vi "PC_SetSelectResistorTo_PLC.vi"(0 "VISA resource name":refnum<visa-resource-name>, 1 "Mode":enum16{"RTU", "ASCII"}(ring), 2 "PLC Address":u8, 3 "Resistor":i32, 5 "error in (no error)":errorcluster) -> (6 "VISA resource name out":refnum<visa-resource-name>, 8 "error out":errorcluster)   [LabVIEW 2015]
panel:
  out "Array":i32[](array[numeric])
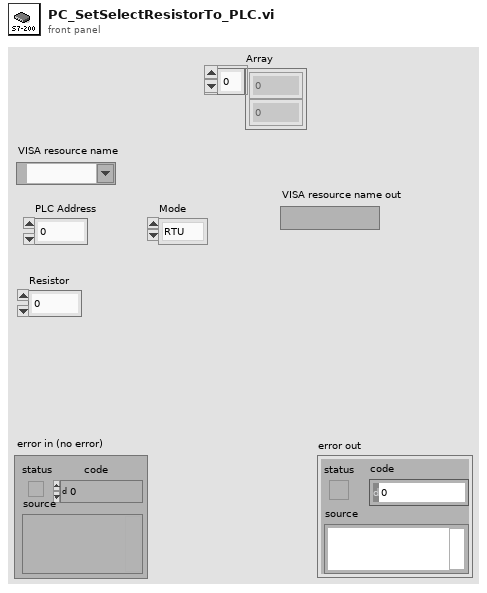
[diagram p1: front panel]
types:
  T1 = cluster{"Mode":enum16{"RTU", "ASCII"}, "Slave Address":u8}
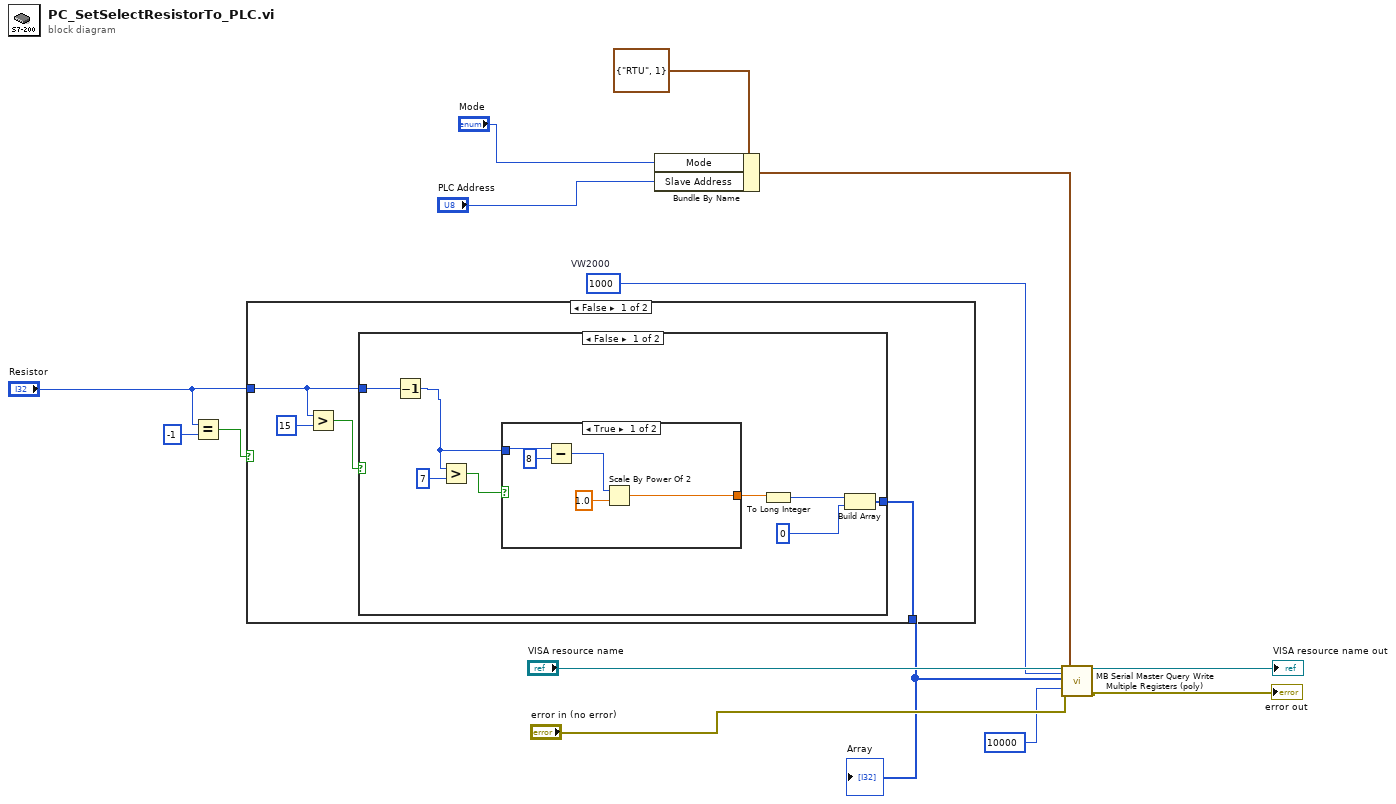
[diagram p0: block diagram]
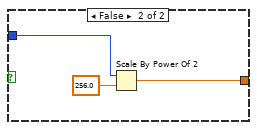
[diagram p2: hidden frame]
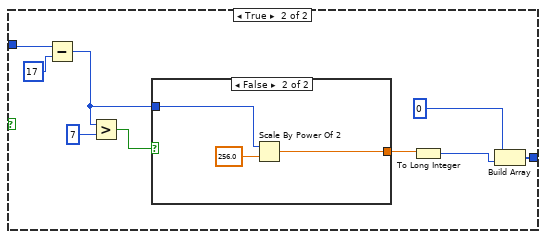
[diagram p3: hidden frame]
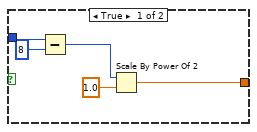
[diagram p4: hidden frame]
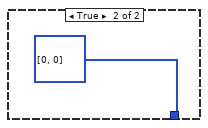
[diagram p5: hidden frame]
diagram:
  w5 = u16 1000  # VW2000
  n1 = Equal?(x="Resistor", y=-1) -> (x = y?=w2:bool)
  n2 = case shown="False" w2 {
    tunnel: "Resistor" -> [w16 _]
    tunnel: [w15 i32[] [0, 0]] -> w4
    frame False {
      n3 = Greater?(x=w16, y=15) -> (0:w17:bool)
      n4 = case shown="False" w17 {
        tunnel: w16 -> [w20 w37]
        tunnel: [w21 w40] -> w15
        frame False {
          n5 = Decrement(x=w20) -> (x-1=w19:i32)
          n6 = Greater?(x=w19, y=7) -> (0:w25:bool)
          n7 = case shown="True" w25 {
            tunnel: w19 -> [w29 w33]
            tunnel: [w30 w32] -> w24
            frame True {
              n8 = Subtract(x=w29, y=8) -> (x-y=w27:i32)
              n9 = Scale By Power Of 2(n=w27, x=1.0) -> (x*2^n=w30:dbl)
            }
            frame False {
              n10 = Scale By Power Of 2(n=w33, x=256.0) -> (x*2^n=w32:dbl)
            }
          }
          n11 = To Long Integer(number=w24) -> (32bit integer=w23:i32)
          n12 = Build Array(w23, 0) -> (w21:i32[])
        }
        frame True {
          n13 = Subtract(x=w37, y=17) -> (x-y=w35:i32)
          n14 = Greater?(x=w35, y=7) -> (0:w42:bool)
          n15 = case shown="False" w42 {
            tunnel: w35 -> [w46 w50]
            tunnel: [w47 w49] -> w41
            frame True {
              n16 = Subtract(x=w46, y=8) -> (x-y=w44:i32)
              n17 = Scale By Power Of 2(n=w44, x=1.0) -> (x*2^n=w47:dbl)
            }
            frame False {
              n18 = Scale By Power Of 2(n=w50, x=256.0) -> (x*2^n=w49:dbl)
            }
          }
          n19 = To Long Integer(number=w41) -> (32bit integer=w39:i32)
          n20 = Build Array(0, w39) -> (w40:i32[])
        }
      }
    }
    frame True {
    }
  }
  "Array" <- w4
  n21 = Bundle By Name(cluster=T1 {"Mode"=enum."RTU", "Slave Address"=1} ("Serial Parameters"), "Mode"="Mode", "Slave Address"="PLC Address") -> (w8:T1)
  n22 = call "MB Serial Master Query Write Multiple Registers (poly).vi"("VISA resource name"="VISA resource name", "Starting Address"=w5, "Registers"=w4, "Timeout"=u32 10000, "error in"="error in (no error)", "Serial Parameters"=w8) -> ("VISA resource name out"=→"VISA resource name out":refnum<visa-resource-name>, "error out"=→"error out":errorcluster)  [unwired: 11 in, 1 out]
